vi "S7 Read.vi"(6 "Data Type":enum16{"I", "Q", "M", "D", "Count", "Timer"}(ring), 7 "DB.NO.":u16, 8 "Error In":errorcluster, 9 "count":u16, 10 "StartByteAddr":u16, 11 "TCP In":refnum<k5>) -> (0 "error out":errorcluster caption="Error Out", 1 "Delay":u32, 2 "Read Data":u8[](array[numeric]), 3 "TCP Out":refnum<k5>)   [LabVIEW 2020]
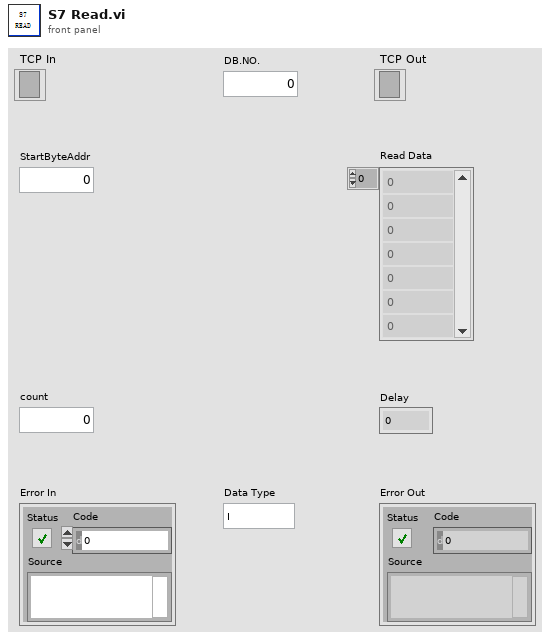
[diagram p1: front panel]
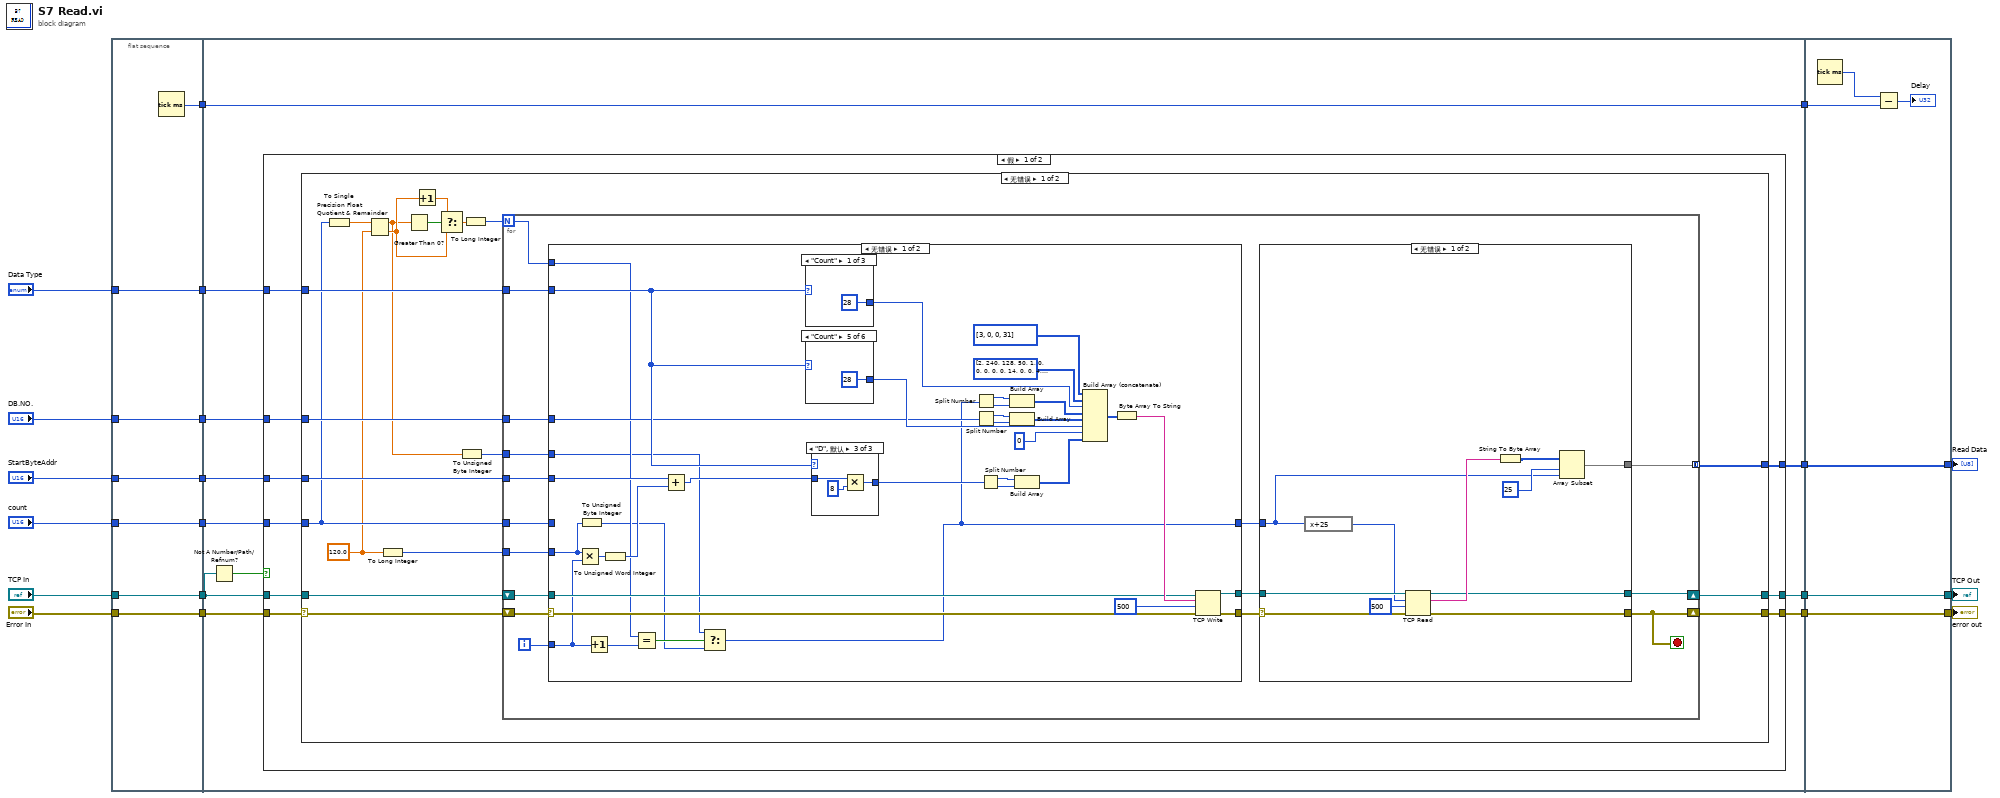
[diagram p0: block diagram]
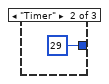
[diagram p5: hidden frame]
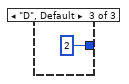
[diagram p6: hidden frame]
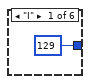
[diagram p7: hidden frame]
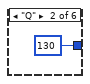
[diagram p8: hidden frame]
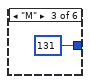
[diagram p9: hidden frame]
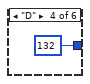
[diagram p10: hidden frame]
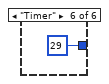
[diagram p11: hidden frame]
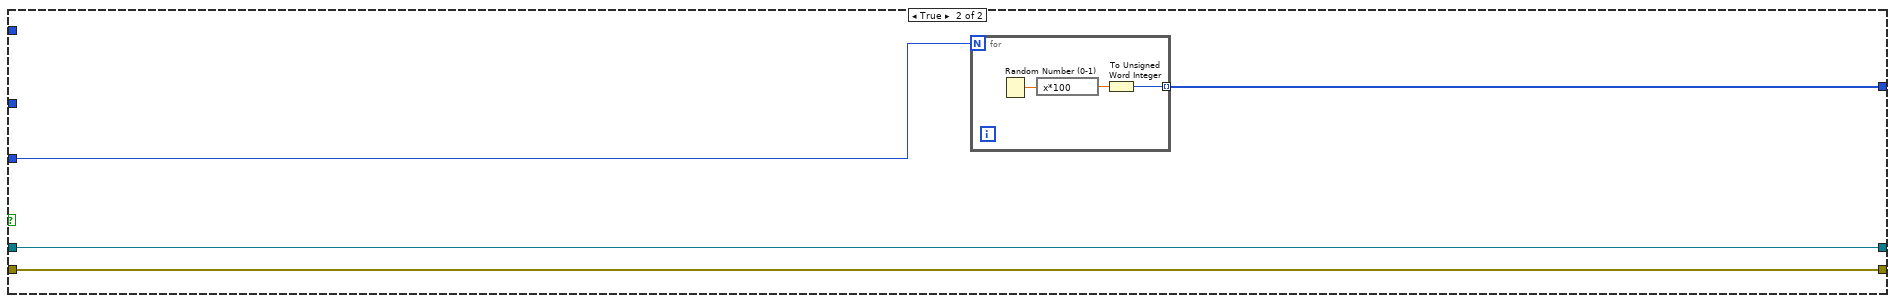
[diagram p14: hidden frame]
diagram:
  n1 = flat-sequence {
    tunnel: "TCP In" -> [w22]
    tunnel: "DB.NO." -> [w23]
    tunnel: "Data Type" -> [w24]
    tunnel: "StartByteAddr" -> [w25]
    tunnel: "Error In" -> [w26]
    tunnel: "count" -> [w27]
    tunnel: [w27] -> w8
    tunnel: [w26] -> w7
    tunnel: [w25] -> w6
    tunnel: [w24] -> w5
    tunnel: [w23] -> w4
    tunnel: [w22] -> w3
    tunnel: [w21] -> w2
    tunnel: [w38] -> w11
    tunnel: [w36] -> w10
    tunnel: [w32] -> w9
    tunnel: w8 -> [w37]
    tunnel: w7 -> [w35]
    tunnel: w6 -> [w34]
    tunnel: w5 -> [w33]
    tunnel: w4 -> [w31]
    tunnel: w3 -> [w30]
    tunnel: w2 -> [w28]
    tunnel: [w28] -> w1
    tunnel: [w161] -> w14
    tunnel: [w162] -> w18
    tunnel: [w163] -> w20
    tunnel: w11 -> [w163]
    tunnel: w10 -> [w162]
    tunnel: w9 -> [w161]
    tunnel: w1 -> [w159]
    frame #0 {
      n2 = Tick Count (ms)() -> (millisecond timer value=w21:u32)
    }
    frame #1 {
      n3 = Not A Number/Path/Refnum?(number/path/refnum=w30) -> (NaN/Path/Refnum?=w29:bool)
      n4 = case shown="假" w29 {
        tunnel: [w47 w154] -> w38
        tunnel: w37 -> [w46 w152]
        tunnel: [w45 w153] -> w36
        tunnel: w35 -> [w44 w153]
        tunnel: w34 -> [w43 _]
        tunnel: w33 -> [w42 _]
        tunnel: [w41 w151] -> w32
        tunnel: w31 -> [w40 _]
        tunnel: w30 -> [w39 w154]
        frame False {
          n5 = case shown="无错误" w44 {
            selector: w44 -> [w65 w149]
            tunnel: [w66 w149] -> w45
            tunnel: w39 -> [w64 w150]
            tunnel: [w63 w150] -> w47
            tunnel: w46 -> [w56 _]
            tunnel: w43 -> [w62 _]
            tunnel: w42 -> [w61 _]
            tunnel: [w60 _] -> w41
            tunnel: w40 -> [w59 _]
            frame No Error {
              w55 = sgl 120.0 ("y")
              n6 = To Single Precision Float(number=w56) -> (single precision float=w50:sgl)
              n7 = Quotient & Remainder(x=w50, y=w55) -> (x-y*floor(x/y)=w49:sgl, floor(x/y)=w51:sgl)
              n8 = To Long Integer(number=w55) -> (32bit integer=w58:i32)
              n9 = Greater Than 0?(x=w49) -> (x > 0?=w54:bool)
              n10 = Increment(x=w51) -> (x+1=w53:sgl)
              n11 = Select(t=w53, s=w54, f=w51) -> (s? t:f=w52:sgl)
              n12 = To Unsigned Byte Integer(number=w49) -> (unsigned 8bit integer=w48:u8)
              n13 = To Long Integer(number=w52) -> (32bit integer=w57:i32)
              n14 = for {
                N: w57 -> [w68]
                tunnel: w62 -> [w76]
                tunnel: w61 -> [w75]
                tunnel: [w74] -> w60 mode=concatenating
                tunnel: w59 -> [w73]
                tunnel: w56 -> [w72]
                shift-right: [w71] -> w66
                shift-left: w65 -> [w80]
                shift-right: [w78] -> w63
                shift-left: w64 -> [w79]
                tunnel: w58 -> [w69]
                tunnel: w48 -> [w67]
                i -> [w70]
                stop <- w71 stop-if-true
                n15 = case shown="无错误" w80 {
                  selector: w80 -> [w111 w147]
                  tunnel: [w114 w148] -> w82
                  tunnel: [w113 w147] -> w77
                  tunnel: [w96 w146] -> w81
                  tunnel: w79 -> [w110 w148]
                  tunnel: w72 -> [_ w146]
                  tunnel: w76 -> [w106 _]
                  tunnel: w75 -> [w109 _]
                  tunnel: w73 -> [w108 _]
                  tunnel: w70 -> [w102 _]
                  tunnel: w69 -> [w103 _]
                  tunnel: w68 -> [w100 _]
                  tunnel: w67 -> [w98 _]
                  frame No Error {
                    n16 = Multiply(x=w103, y=w102) -> (x*y=w107:i32)
                    n17 = To Unsigned Byte Integer(number=w103) -> (unsigned 8bit integer=w97:u8)
                    n18 = Increment(x=w102) -> (x+1=w101:i32)
                    n19 = To Unsigned Word Integer(number=w107) -> (unsigned 16bit integer=w104:u16)
                    n20 = Equal?(x=w100, y=w101) -> (x = y?=w99:bool)
                    n21 = Add(x=w106, y=w104) -> (x+y=w105:u16)
                    n22 = Select(t=w98, s=w99, f=w97) -> (s? t:f=w96:u8)
                    n23 = case shown="\"Count\"" w109 {
                      tunnel: [u8 28 ("DB.NO. 3") u8 29 ("DB.NO. 3") u8 2 ("DB.NO. 3")] -> w119
                      frame "Count" {
                      }
                      frame "Timer" {
                      }
                      frame "D", Default {
                      }
                    }
                    n24 = case shown="\"Count\"" w109 {
                      tunnel: [u8 129 ("DB.NO. 3") u8 130 ("DB.NO. 3") u8 131 ("DB.NO. 3") u8 132 ("DB.NO. 3") u8 28 ("DB.NO. 3") u8 29 ("DB.NO. 3")] -> w124
                      frame "I" {
                      }
                      frame "Q" {
                      }
                      frame "M" {
                      }
                      frame "D" {
                      }
                      frame "Count" {
                      }
                      frame "Timer" {
                      }
                    }
                    n25 = case shown="\"D\", 默认" w109 {
                      tunnel: [w132 w133 w135] -> w118
                      tunnel: w105 -> [w132 w133 w136]
                      frame "Count" {
                      }
                      frame "Timer" {
                      }
                      frame "D", Default {
                        n26 = Multiply(x=w136, y=u16 8) -> (x*y=w135:u16)
                      }
                    }
                    n27 = Split Number(x=w96) -> (hi(x)=w127:u8, lo(x)=w128:u8)
                    n28 = Split Number(x=w108) -> (hi(x)=w126:u8, lo(x)=w125:u8)
                    n29 = Split Number(x=w118) -> (hi(x)=w117:u8, lo(x)=w116:u8)
                    n30 = Build Array(w127, w128) -> (w121:u8[])
                    n31 = Build Array(w126, w125) -> (w122:u8[])
                    n32 = Build Array(w117, w116) -> (w115:u8[])
                    n33 = Build Array (concatenate)(u8[] [3, 0, 0, 31], u8[] [2, 240, 128, 50, 1, 0, 0, 0, 0, 0, 14, 0, 0, 4, 1, 18, 10, 16], w119, w121, w122, w124, u8 0 ("DB.NO. 3"), w115) -> (w120:u8[])
                    n34 = Byte Array To String(unsigned byte array=w120) -> (string=w131:string)
                    n35 = TCP Write(connection ID=w110, data in=w131, error in (no error)=w111, 9:500 ("timeout ms (25000)")) -> (connection ID out=w114:refnum<k5>, error out=w113:errorcluster)  [unwired: 1 out]
                  }
                  frame Error {
                  }
                }
                n36 = case shown="无错误" w77 {
                  selector: w77 -> [w85 w94]
                  tunnel: w82 -> [w93 w95]
                  tunnel: w81 -> [w88 _]
                  tunnel: [w83 w94] -> w71
                  tunnel: [w86 w95] -> w78
                  tunnel: [w84 _] -> w74
                  frame No Error {
                    n37 = expression code="x+25"(w88) -> (w92:u16)
                    n38 = TCP Read(connection ID=w93, bytes to read=w92, error in (no error)=w85, 9:500 ("timeout ms (25000)")) -> (connection ID out=w86:refnum<k5>, data out=w91:string, error out=w83:errorcluster)  [unwired: 1 in]
                    n39 = String To Byte Array(string=w91) -> (unsigned byte array=w90:u8[])
                    n40 = Array Subset(array=w90, index=25, length=w88) -> (w84:u8[])
                  }
                  frame Error {
                  }
                }
              }
            }
            frame Error {
            }
          }
        }
        frame True {
          n41 = for {
            N: w152 -> [_]
            tunnel: [w155] -> w151 mode=indexing
            n42 = Random Number (0-1)() -> (number: 0 to 1=w157:dbl)
            n43 = expression code="x*100"(w157) -> (w156:dbl)
            n44 = To Unsigned Word Integer(number=w156) -> (unsigned 16bit integer=w155:u16)
          }
        }
      }
    }
    frame #2 {
      n45 = Tick Count (ms)() -> (millisecond timer value=w160:u32)
      n46 = Subtract(x=w160, y=w159) -> (x-y=→"Delay":u32)
    }
  }
  "TCP Out" <- w20
  "error out" <- w18
  "Read Data" <- w14
